vi "Recursive Child Symbol Reader.vi"(8 "error in (no error)":errorcluster, 9 ".NET TcAdsSymbolInfo":refnum<k24>, 11 "TwinCAT ADS in":refnum<class "TwinCAT ADS.lvclass">) -> (0 "error out":errorcluster, 1 "Symbols Information":T1[](array[typedef]) {"Type ID" items=["ADST_VOID"=0, "ADST_INT16"=2, "ADST_INT32"=3, "ADST_REAL32"=4, "ADST_REAL64"=5, "ADST_INT8"=16, "ADST_UINT8"=17, "ADST_UINT16"=18, "ADST_UINT32"=19, "ADST_INT64"=20, "ADST_UINT64"=21, "ADST_STRING"=30, "ADST_WSTRING"=31, "ADST_REAL80"=32, "ADST_BIT"=33, "ADST_MAXTYPES"=34, "ADST_BIGTYPE"=65]; "Type Category" items=["Unknown, None"=0, "Primitive"=1, "Alias"=2, "Enum"=3, "Array"=4, "Struct"=5, "FunctionBlock"=6, "Program"=7, "Function"=8, "SubRange"=9, "String"=10, "Bitset"=12, "Pointer"=13, "Union"=14, "Reference"=15, "Interface"=16]}, 3 "TwinCAT ADS out":refnum<class "TwinCAT ADS.lvclass">)   [LabVIEW 2018, in "TwinCAT ADS.lvclass"]
uses:
  TwinCAT ADS.lvclass
  TwinCAT.Ads
  Controls/Symbol Information.ctl
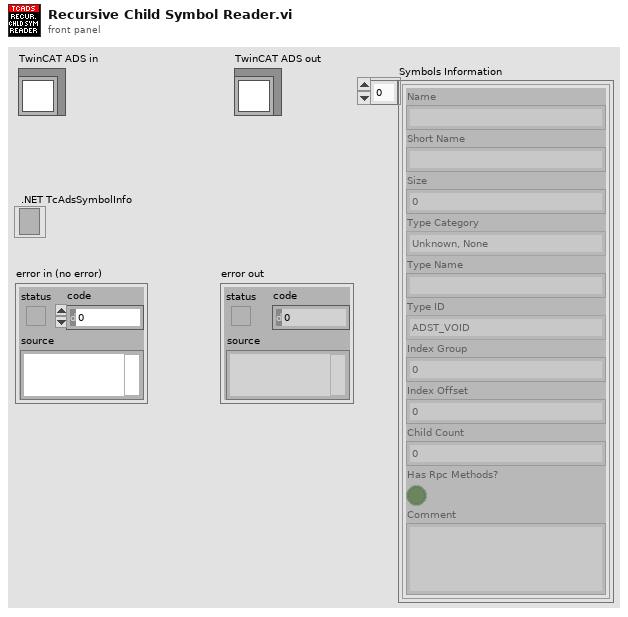
[diagram p1: front panel]
types:
  T1 = typedef "TwinCAT ADS.lvclass/Symbol Information.ctl" = cluster{"Name":string, "Short Name":string, "Size":i32, "Type Category":i32, "Type Name":string, "Type ID":i32, "Index Group":i64, "Index Offset":i64, "Child Count":i32, "Has Rpc Methods?":bool, "Comment":string}
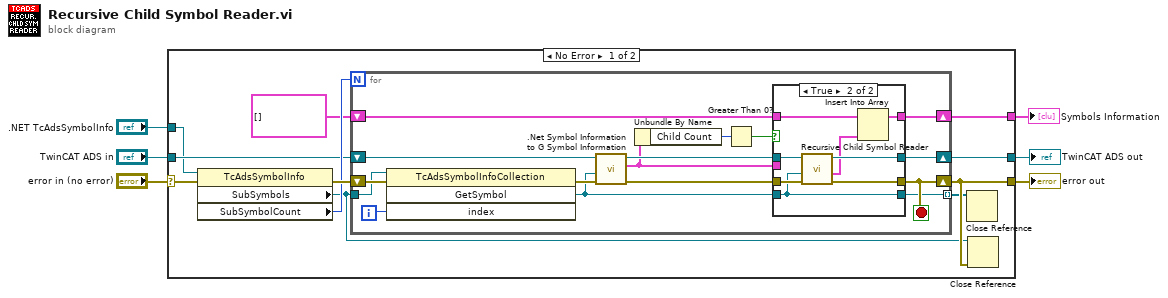
[diagram p0: block diagram]
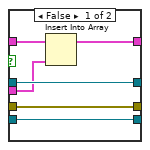
[diagram p2: hidden frame]
diagram:
  n1 = case shown="No Error" "error in (no error)" {
    selector: "error in (no error)" -> [w14 w49]
    tunnel: [w9 w49] -> w5
    tunnel: [w12 w48] -> w3
    tunnel: "TwinCAT ADS in" -> [w15 w48]
    tunnel: ".NET TcAdsSymbolInfo" -> [w13 _]
    tunnel: [w10 _] -> w1
    frame No Error {
      n2 = property class="TcAdsSymbolInfo"(reference=w13, error in=w14) -> (error out=w17:errorcluster, "SubSymbols"=w7:refnum<k24>, "SubSymbolCount"=w16:i32)  [unwired: 1 out]
      n3 = for {
        N: w16 -> [_]
        tunnel: w7 -> [w32]
        shift-right: [w19] -> w9
        shift-left: w17 -> [w33]
        shift-right: [w20] -> w10
        shift-left: T1[] [] -> [w21]
        shift-right: [w22] -> w12
        shift-left: w15 -> [w29]
        tunnel: [w18] -> w8 mode=indexing
        i -> [w31]
        stop <- w19 stop-if-true
        n4 = invoke class="TcAdsSymbolInfoCollection" method="GetSymbol"(reference=w32, error in=w33, "index"=w31) -> (error out=w30:errorcluster, "GetSymbol"=w24:refnum<k24>)  [unwired: 1 in, 2 out]
        n5 = call ".Net Symbol Information to G Symbol Information.vi"("TwinCAT ADS in"=w29, ".NET AdsSymbolInfo"=w24, "error in (no error)"=w30) -> ("TwinCAT ADS out"=w26:refnum<class "TwinCAT ADS.lvclass">, "Symbol Information"=w23:T1, "error out"=w25:errorcluster)  [unwired: 5 in]
        n6 = Unbundle By Name(w23) -> ("Child Count"=w28:i32)
        n7 = Greater Than 0?(x=w28) -> (x > 0?=w27:bool)
        n8 = case shown="True" w27 {
          tunnel: w26 -> [w39 w46]
          tunnel: w25 -> [w38 w47]
          tunnel: w24 -> [w34 w40]
          tunnel: w23 -> [w35 _]
          tunnel: [w39 w44] -> w22
          tunnel: [w38 w45] -> w19
          tunnel: w21 -> [w37 w43]
          tunnel: [w36 w42] -> w20
          tunnel: [w34 w40] -> w18
          frame False {
            n9 = Insert Into Array(array=w37, new element=w35) -> (w36:T1[])  [unwired: 1 in]
          }
          frame True {
            n10 = call "Recursive Child Symbol Reader.vi"("error in (no error)"=w47, ".NET TcAdsSymbolInfo"=w40, "TwinCAT ADS in"=w46) -> ("error out"=w45:errorcluster, "Symbols Information"=w41:T1[], "TwinCAT ADS out"=w44:refnum<class "TwinCAT ADS.lvclass">)  [unwired: 6 in]
            n11 = Insert Into Array(array=w43, new element=w41) -> (w42:T1[])  [unwired: 1 in]
          }
        }
      }
      n12 = Close Reference(reference=w8) -> ()  [unwired: 1 in, 1 out]
      n13 = Close Reference(reference=w7, error in (no error)=w9) -> ()  [unwired: 1 out]
    }
    frame Error {
    }
  }
  "error out" <- w5
  "TwinCAT ADS out" <- w3
  "Symbols Information" <- w1
